vi "Read File.vi"(8 "error in (no error)":errorcluster, 10 "Path":path) -> (0 "error out":errorcluster, 3 "json class out":refnum<class "json class.lvclass">)   [LabVIEW 2021, in "Config Library.lvlib" / "json class.lvclass"]
uses:
  json class.lvclass
  json class.lvclass/json class.ctl
  <vilib>/addons/JSON API/JSON Value/Set from JSON string.vi
  <vilib>/addons/JSON API/JSON Value/JSON Value.lvclass
  <vilib>/addons/JSON API/Get Polymorphic/JSON GetSet.lvlib
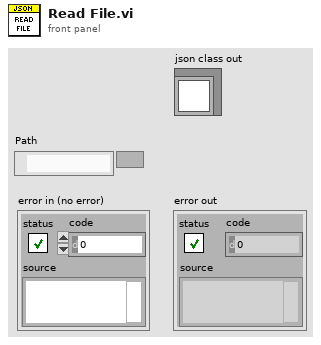
[diagram p1: front panel]
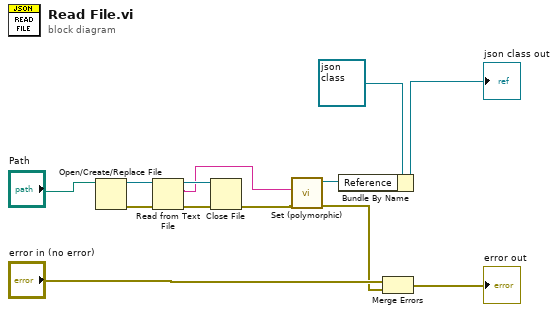
[diagram p0: block diagram]
diagram:
  n1 = Open/Create/Replace File(file path (use dialog)="Path") -> (refnum out=w12:refnum<file>, error out=w9:errorcluster)  [unwired: 5 in, 1 out]
  n2 = Read from Text File(file (use dialog)=w12, error in=w9) -> (refnum out=w11:refnum<file>, text=w7:string, error out=w10:errorcluster)  [unwired: 2 in, 1 out]
  n3 = Close File(refnum=w11, error in=w10) -> (error out=w8:errorcluster)  [unwired: 1 out]
  n4 = call-poly <vilib>:"Set (polymorphic).vi"("error in (no error)"=w8, "JSON stream"=w7) -> ("error out"=w1:errorcluster, "JSON Value out"=w4:refnum<class "JSON Value.lvclass">)  [unwired: 7 in, 1 out]
  n5 = Bundle By Name(cluster=refnum<class "json class.lvclass"> refnum ("json class in"), "Reference"=w4) -> (→"json class out":refnum<class "json class.lvclass">)
  n6 = Merge Errors("error in (no error)", w1) -> (→"error out":errorcluster)
